vi "test Parse Sorted Object Dictionary_5.vi"(11 "Test Case In":refnum<class "test EDS.lvclass">) -> (0 "error out":errorcluster, 3 "Test Case Out":refnum<class "test EDS.lvclass">)   [LabVIEW 2024, in "test EDS.lvclass"]
uses:
  test EDS.lvclass
  C:/Program Files/National Instruments/LabVIEW 2024/vi.lib/Astemes/LUnit/Test Case.lvclass
  Core/EDS/EDS.lvclass
  Core/EDS/EDS.lvclass/EDS.ctl
  <vilib>/Astemes/LUnit/Test Case.lvclass/Test Case.ctl
  997a5cc8-28e7-4c8b-bc0c-c7deaea17f55.vi
  <vilib>/Astemes/LUnit/Append Pass Result.vi
  <vilib>/Astemes/LUnit/Append Fail Result.vi
  <vilib>/Astemes/LUnit/Describe Comparison.vi
  997a5cc8-28e7-4c8b-bc0c-c7deaea17f55.vi/9c5d11cd-9439-4240-a1ee-d9baace9c924.vi
  <vilib>/Astemes/LUnit/Run In UI.vi
  <vilib>/Utility/error.llb/Clear Errors.vi
  <vilib>/Astemes/LUnit/Describe Variant.vi
  Core/OD Entry/OD Entry.lvclass
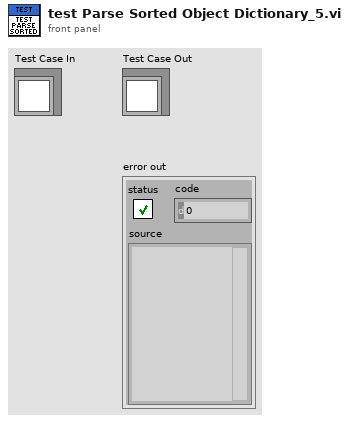
[diagram p1: front panel]
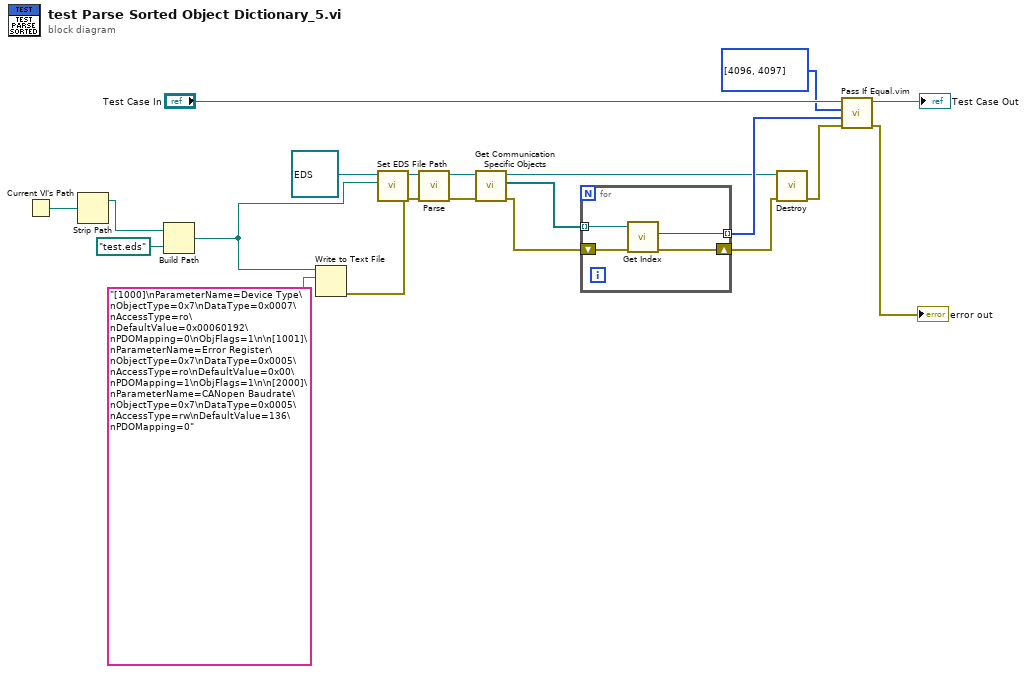
[diagram p0: block diagram]
diagram:
  n1 = Current VI's Path() -> (path=w15:path)
  n2 = Strip Path(path=w15) -> (stripped path=w11:path)  [unwired: 1 out]
  n3 = Build Path(base path=w11, name or relative path=path "test.eds") -> (appended path=w12:path)
  n4 = Write to Text File(file (use dialog)=w12, text="[1000]\nParameterName=Device Type\nObjectType=0x7\nDataType=0x0007\nAccessType=ro\nDefaultValue=0x00060192\nPDOMapping=0\nObjFlags=1\n\n[1001]\nParameterName=Error Register\nObjectType=0x7\nDataType=0x0005\nAccessType=ro\nDefaultValue=0x00\nPDOMapping=1\nObjFlags=1\n\n[2000]\nParameterName=CANopen Baudrate\nObjectType=0x7\nDataType=0x0005\nAccessType=rw\nDefaultValue=136\nPDOMapping=0") -> (error out=w13:errorcluster)  [unwired: 2 in, 2 out]
  n5 = call "Set EDS File Path.vi"("EDS File Path"=w12, "EDS in"=refnum<class "EDS.lvclass"> refnum ("EDS.lvlib:EDS.lvclass")) -> ("EDS out"=w16:refnum<class "EDS.lvclass">)  [unwired: 9 in]
  n6 = call "Parse.vi"("error in"=w13, "EDS in"=w16) -> ("error out"=w8:errorcluster, "EDS out"=w4:refnum<class "EDS.lvclass">)  [unwired: 8 in]
  n7 = call "Get Communication Specific Objects.vi"("error in"=w8, "EDS in"=w4) -> ("error out"=w2:errorcluster, "Entries"=w7:refnum<class "OD Entry.lvclass">[], "EDS out"=w3:refnum<class "EDS.lvclass">)  [unwired: 7 in]
  n8 = for {
    tunnel: w7 -> [w24] mode=indexing
    tunnel: [w23] -> w5 mode=indexing
    shift-right: [w21] -> w1
    shift-left: w2 -> [w22]
    n9 = call "Get Index.vi"("Error In"=w22, "reference in"=w24) -> ("Error Out"=w21:errorcluster, "Index"=w23:u16)  [unwired: 7 in, 1 out]
  }
  n10 = call "Destroy.vi"("error in"=w1, "EDS in"=w3) -> ("error out"=w9:errorcluster)  [unwired: 8 in, 1 out]
  n11 = call "Pass If Equal.vim"("error in (no error)"=w9, "Actual"=w5, "Expected"=u16[] [4096, 4097] ("Array"), "LUnit Test Case In"="Test Case In") -> ("error out"=→"error out":errorcluster, "LUnit Test Case Out"=→"Test Case Out":refnum<class "test EDS.lvclass">)  [unwired: 6 in]
